vi "Image Display Save Overlay.vi"(8 "error in (no error)":errorcluster, 9 "Saved Image File Format":T2, 10 "File Path in":path, 11 "Display Image Control Refnum":T1) -> (0 "Error Out":errorcluster, 2 "File Path out":path)   [LabVIEW 2021, in "Image.lvlib"]
uses:
  Image Save File Format.ctl
  Image Control Refnum.ctl
  Image.lvlib
  Error/Error.lvlib
  <vilib>/vision/NI_Vision_Development_Module.lvlib
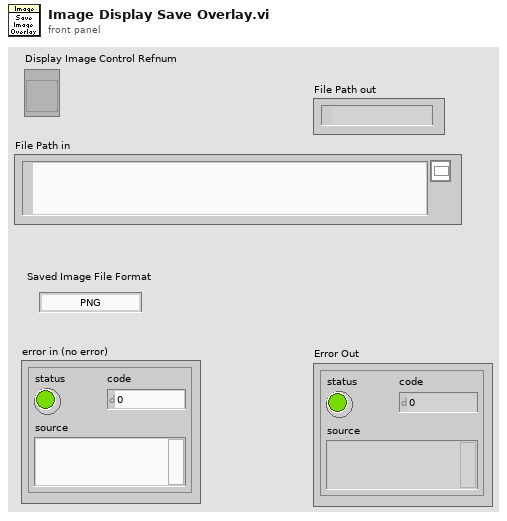
[diagram p1: front panel]
types:
  T1 = typedef "Image.lvlib/Image Control Refnum.ctl" = refnum<vi>
  T2 = typedef "Image.lvlib/Image Save File Format.ctl" = enum16{"PNG", "JPEG", "BMP"}
  T3 = typedef "Image Type" = u32
  T4 = typedef "Color (U64)" = cluster{"Plane 3 (Blue)":u16, "Plane 2 (Green)":u16, "Plane 1 (Red)":u16, "Plane 4 (alpha)":u16}
  T5 = typedef "IMAQ Image.ctl" = refnum<image>
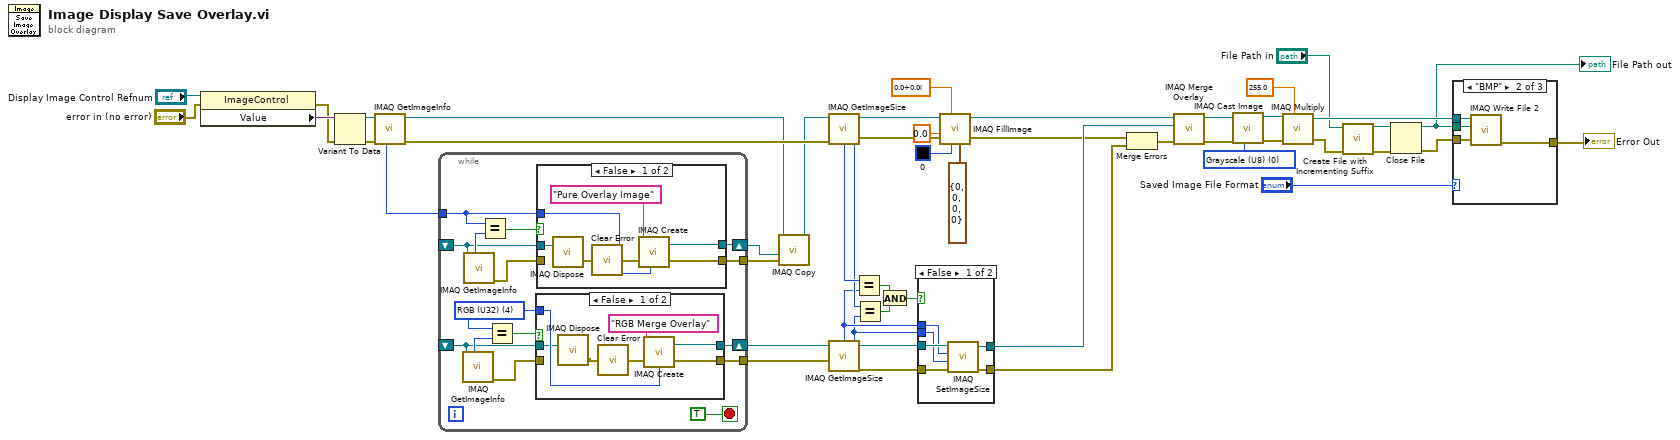
[diagram p0: block diagram]
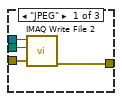
[diagram p2: hidden frame]
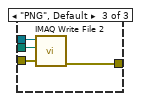
[diagram p3: hidden frame]
diagram:
  w13 = T3 0 items=["Grayscale (U8)", "Grayscale (I16)", "Grayscale (SGL)", "Complex (CSG)", "RGB (U32)", "HSL (U32)", "RGB (U64)", "Grayscale (U16)"] ("Image Type")
  n1 = property class="ImageControl"(reference="Display Image Control Refnum", error in="error in (no error)") -> (error out=w44:errorcluster, "Value"=w45:variant)  [unwired: 1 out]
  n2 = Variant To Data(error in=w44, Variant=w45) -> (data=w26:T5, error out=w31:errorcluster)  [unwired: 1 in]
  n3 = call "IMAQ GetImageInfo"("error in (no error)"=w31, "Image"=w26) -> ("error out"=w30:errorcluster, "Image Type"=w29:T3)  [unwired: 2 in, 6 out]
  n4 = while {
    shift-right: [w56] -> w35
    shift-left: _ -> [w55]
    tunnel: [w54] -> w41
    shift-right: [w50] -> w28
    shift-left: _ -> [w49]
    tunnel: w29 -> [w51]
    tunnel: [w48] -> w27
    stop <- TRUE stop-if-true
    w57 = T3 4 items=["Grayscale (U8)", "Grayscale (I16)", "Grayscale (SGL)", "Complex (CSG)", "RGB (U32)", "HSL (U32)", "RGB (U64)", "Grayscale (U16)"] ("Image Type")
    n5 = call "IMAQ GetImageInfo"("Image"=w55) -> ("error out"=w58:errorcluster, "Image Type"=w60:T3)  [unwired: 3 in, 6 out]
    n6 = call "IMAQ GetImageInfo"("Image"=w49) -> ("error out"=w47:errorcluster, "Image Type"=w53:T3)  [unwired: 3 in, 6 out]
    n7 = Equal?(x=w51, y=w53) -> (x = y?=w52:bool)
    n8 = Equal?(x=w57, y=w60) -> (x = y?=w59:bool)
    n9 = case shown="False" w59 {
      tunnel: w58 -> [_ w79]
      tunnel: [w75 w78] -> w56
      tunnel: w57 -> [w76 _]
      tunnel: [w74 w79] -> w54
      tunnel: w55 -> [w73 w78]
      frame False {
        n10 = call "IMAQ Dispose"("Image"=w73) -> ("error out"=w72:errorcluster)  [unwired: 5 in]
        n11 = call "Clear Error.vi"("Error In"=w72) -> ("no Error Out"=w71:errorcluster)  [unwired: 8 in]
        n12 = call "IMAQ Create"("Image Name"="RGB Merge Overlay", "Image Type"=w76, "error in (no error)"=w71) -> ("New Image"=w75:T5, "error out"=w74:errorcluster)  [unwired: 2 in]
      }
      frame True {
      }
    }
    n13 = case shown="False" w52 {
      tunnel: w51 -> [w68 _]
      tunnel: [w66 w70] -> w50
      tunnel: w49 -> [w65 w70]
      tunnel: [w62 w69] -> w48
      tunnel: w47 -> [_ w69]
      frame False {
        n14 = call "IMAQ Dispose"("Image"=w65) -> ("error out"=w64:errorcluster)  [unwired: 5 in]
        n15 = call "Clear Error.vi"("Error In"=w64) -> ("no Error Out"=w63:errorcluster)  [unwired: 8 in]
        n16 = call "IMAQ Create"("Image Name"="Pure Overlay Image", "Image Type"=w68, "error in (no error)"=w63) -> ("New Image"=w66:T5, "error out"=w62:errorcluster)  [unwired: 2 in]
      }
      frame True {
      }
    }
  }
  n17 = call "IMAQ Copy"("error in (no error)"=w27, "Image Dst"=w28, "Image Src"=w26) -> ("Image Dst Out"=w23:T5)  [unwired: 3 in, 1 out]
  n18 = call "IMAQ GetImageSize"("Image"=w23, "error in (no error)"=w30) -> ("Y Resolution"=w39:i32, "X Resolution"=w40:i32, "error out"=w22:errorcluster)  [unwired: 2 in]
  n19 = call "IMAQ GetImageSize"("Image"=w35, "error in (no error)"=w41) -> ("Y Resolution"=w32:i32, "X Resolution"=w33:i32, "error out"=w34:errorcluster)  [unwired: 2 in]
  n20 = Equal?(x=w40, y=w33) -> (x = y?=w38:bool)
  n21 = Equal?(x=w39, y=w32) -> (x = y?=w37:bool)
  n22 = And(x=w38, y=w37) -> (x .and. y?=w36:bool)
  n23 = case shown="False" w36 {
    tunnel: w35 -> [w85 w87]
    tunnel: w34 -> [w84 w86]
    tunnel: w33 -> [w83 _]
    tunnel: w32 -> [w82 _]
    tunnel: [w81 w87] -> w25
    tunnel: [w80 w86] -> w24
    frame False {
      n24 = call "IMAQ SetImageSize"("error in (no error)"=w84, "Y Resolution"=w82, "X Resolution"=w83, "Image"=w85) -> ("error out"=w80:errorcluster, "Image Out"=w81:T5)  [unwired: 1 in]
    }
    frame True {
    }
  }
  n25 = call "IMAQ FillImage"("Color (U64)"=T4 {"Plane 3 (Blue)"=0, "Plane 2 (Green)"=0, "Plane 1 (Red)"=0, "Plane 4 (alpha)"=0}, "Color Pixel Value"=u32 0, "Complex Pixel Value"=csg 0.0+0.0i, "error in (no error)"=w22, "Pixel Value (U8, U16, I16, Float)"=sgl 0.0, "Image"=w23) -> ("error out"=w20:errorcluster, "Image Out"=w21:T5)  [unwired: 4 in]
  n26 = Merge Errors(w20, w24) -> (w42:errorcluster)
  n27 = call "IMAQ Merge Overlay"("error in (no error)"=w42, "Image Dst"=w25, "Image Src"=w21) -> ("error out"=w14:errorcluster, "Image Dst Out"=w15:T5)  [unwired: 7 in]
  n28 = call "IMAQ Cast Image"("Image Type"=w13, "error in (no error)"=w14, "Image Src"=w15) -> ("error out"=w11:errorcluster, "Image Dst Out"=w12:T5)  [unwired: 7 in]
  n29 = call "IMAQ Multiply"("Image Src A"=w12, "Constant"=255.0, "error in (no error)"=w11) -> ("Image Dst Out"=w9:T5, "error out"=w7:errorcluster)  [unwired: 4 in]
  n30 = call <vilib>:"Create File with Incrementing Suffix.vi"("error in (no error)"=w7, "file path"="File Path in") -> ("error out"=w5:errorcluster, "refnum out"=w3:refnum<file>)  [unwired: 7 in, 1 out]
  n31 = Close File(refnum=w3, error in=w5) -> (path=w2:path, error out=w4:errorcluster)
  "File Path out" <- w2
  n32 = case shown="\"BMP\"" "Saved Image File Format" {
    tunnel: w4 -> [w91 w95 w99]
    tunnel: w9 -> [w90 w94 w98]
    tunnel: w2 -> [w89 w93 w97]
    tunnel: [w88 w92 w96] -> w1
    frame "JPEG" {
      n33 = call-poly "IMAQ Write File 2"("error in (no error)"=w91, "File Path"=w89, "Image"=w90) -> ("error out"=w88:errorcluster)  [unwired: 7 in, 1 out]
    }
    frame "BMP" {
      n34 = call-poly "IMAQ Write File 2"("error in (no error)"=w95, "File Path"=w93, "Image"=w94) -> ("error out"=w92:errorcluster)  [unwired: 7 in, 1 out]
    }
    frame "PNG", Default {
      n35 = call-poly "IMAQ Write File 2"("error in (no error)"=w99, "File Path"=w97, "Image"=w98) -> ("error out"=w96:errorcluster)  [unwired: 7 in, 1 out]
    }
  }
  "Error Out" <- w1
